vi "Pour.vi"(8 "error in (no error)":errorcluster, 11 "Guiness in":refnum<class "Guiness.lvclass">) -> (0 "error out":errorcluster, 3 "Guiness out":refnum<class "Guiness.lvclass">)   [LabVIEW 2011, in "Guiness.lvclass"]
uses:
  Guiness.lvclass
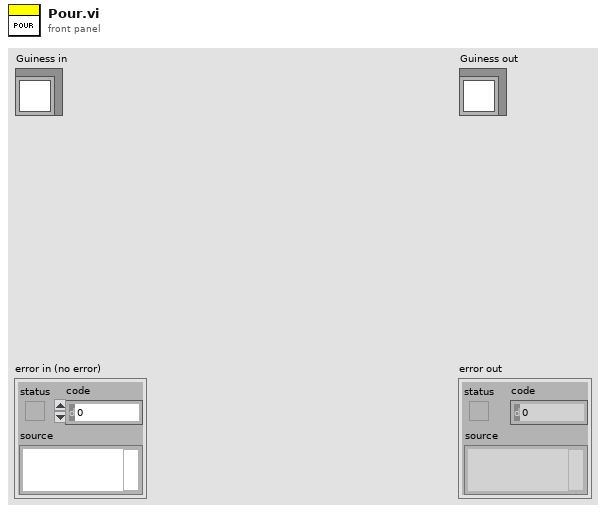
[diagram p1: front panel]
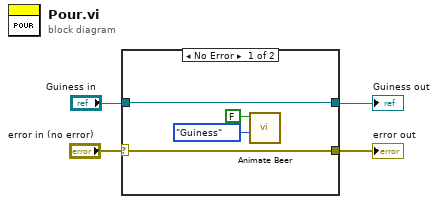
[diagram p0: block diagram]
diagram:
  n1 = case shown="No Error" "error in (no error)" {
    selector: "error in (no error)" -> [w7 w9]
    tunnel: "Guiness in" -> [w8 w10]
    tunnel: [w8 w10] -> w1
    tunnel: [w7 w9] -> w2
    frame No Error {
      n2 = call "Animate Beer.vi"("Type"=enum16{"Lager", "Ale", "Guiness"}."Guiness", "Tilt"=FALSE) -> ()  [unwired: 10 in]
    }
    frame Error {
    }
  }
  "error out" <- w2
  "Guiness out" <- w1
